vi "test_libssh2_channel_write_stderr.vi"() -> ()   [LabVIEW 2013, in "libssh2_integration_tests.lvlib"]
uses:
  libssh2_integration_tests.lvlib
  <vilib>/addons/_JKI Toolkits/Caraya/classes/Test/Test.lvclass
  libssh2/libssh2.lvlib
  <vilib>/addons/_JKI Toolkits/Caraya/classes/Assert/Assert.lvclass
panel:
  out "error out":errorcluster
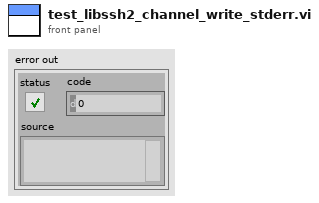
[diagram p1: front panel]
types:
  T1 = typedef "libssh2.lvlib/Session Refnum.ctl" = refnum<k1>
  T2 = typedef "libssh2.lvlib/Channel Refnum.ctl" = refnum<k1>
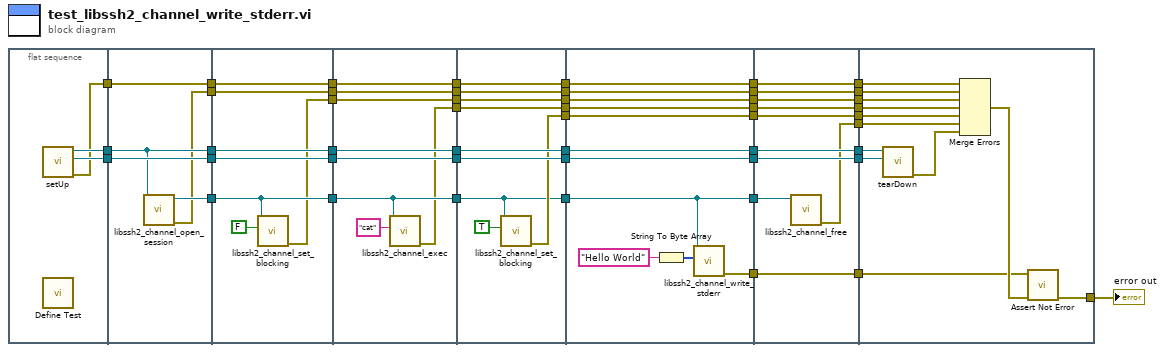
[diagram p0: block diagram]
diagram:
  n1 = flat-sequence {
    tunnel: [w51] -> w48
    tunnel: [w50] -> w47
    tunnel: [w49] -> w46
    tunnel: w48 -> [w55]
    tunnel: w47 -> [w56]
    tunnel: [w55] -> w38
    tunnel: [w56] -> w36
    tunnel: [w54] -> w30
    tunnel: w46 -> [w53]
    tunnel: [w53] -> w34
    tunnel: [w52] -> w32
    tunnel: w38 -> [w63]
    tunnel: [w63] -> w37
    tunnel: w36 -> [w62]
    tunnel: [w62] -> w35
    tunnel: w34 -> [w61]
    tunnel: [w61] -> w33
    tunnel: w32 -> [w60]
    tunnel: [w60] -> w31
    tunnel: w30 -> [w59]
    tunnel: [w59] -> w29
    tunnel: [w57] -> w28
    tunnel: w37 -> [w71]
    tunnel: [w71] -> w26
    tunnel: w35 -> [w70]
    tunnel: [w70] -> w24
    tunnel: w33 -> [w69]
    tunnel: [w69] -> w22
    tunnel: w31 -> [w68]
    tunnel: [w68] -> w20
    tunnel: w29 -> [w67]
    tunnel: [w67] -> w18
    tunnel: [w65] -> w16
    tunnel: w28 -> [w64]
    tunnel: [w64] -> w14
    tunnel: w26 -> [w80]
    tunnel: [w80] -> w25
    tunnel: w24 -> [w79]
    tunnel: [w79] -> w23
    tunnel: w22 -> [w78]
    tunnel: [w78] -> w21
    tunnel: w20 -> [w77]
    tunnel: [w77] -> w19
    tunnel: w18 -> [w72]
    tunnel: [w72] -> w17
    tunnel: w16 -> [w76]
    tunnel: [w76] -> w15
    tunnel: w14 -> [w75]
    tunnel: [w75] -> w13
    tunnel: [w73] -> w12
    tunnel: w25 -> [w91]
    tunnel: [w91] -> w9
    tunnel: w23 -> [w90]
    tunnel: [w90] -> w8
    tunnel: w21 -> [w89]
    tunnel: [w89] -> w7
    tunnel: w19 -> [w88]
    tunnel: [w88] -> w6
    tunnel: w17 -> [w87]
    tunnel: [w87] -> w5
    tunnel: w15 -> [w86]
    tunnel: [w86] -> w4
    tunnel: w13 -> [w85]
    tunnel: [w85] -> w3
    tunnel: w12 -> [w84]
    tunnel: [w84] -> w2
    tunnel: [w83] -> w1
    tunnel: w9 -> [w101]
    tunnel: w8 -> [w100]
    tunnel: [w101] -> w45
    tunnel: [w100] -> w44
    tunnel: [w99] -> w43
    tunnel: w7 -> [w98]
    tunnel: [w98] -> w42
    tunnel: w6 -> [w97]
    tunnel: [w97] -> w41
    tunnel: w5 -> [w96]
    tunnel: w4 -> [w95]
    tunnel: [w95] -> w39
    tunnel: w3 -> [w94]
    tunnel: [w94] -> w27
    tunnel: w2 -> [w93]
    tunnel: [w93] -> w11
    tunnel: [w92] -> w10
    tunnel: w1 -> [w92]
    tunnel: w45 -> [w113]
    tunnel: w44 -> [w112]
    tunnel: [w111] -> w40
    tunnel: w43 -> [w109]
    tunnel: w42 -> [w108]
    tunnel: w41 -> [w106]
    tunnel: w39 -> [w105]
    tunnel: w27 -> [w104]
    tunnel: w11 -> [w103]
    tunnel: w10 -> [w102]
    frame #0 {
      n2 = call "setUp.vi"() -> ("error out"=w49:errorcluster, "connection ID"=w50:refnum<k5>, "session"=w51:T1)  [unwired: 9 in]
      n3 = call <vilib>:"Define Test.vi"() -> ()  [unwired: 10 in, 2 out]
    }
    frame #1 {
      n4 = call "libssh2_channel_open_session.vi"("session"=w55) -> ("error out"=w52:errorcluster, "channel"=w54:T2)  [unwired: 9 in]
    }
    frame #2 {
      n5 = call "libssh2_channel_set_blocking.vi"("blocking"=FALSE, "channel"=w59) -> ("error out"=w57:errorcluster)  [unwired: 9 in]
    }
    frame #3 {
      n6 = call "libssh2_channel_exec.vi"("command"="cat", "channel"=w67) -> ("error out"=w65:errorcluster)  [unwired: 9 in]
    }
    frame #4 {
      n7 = call "libssh2_channel_set_blocking.vi"("blocking"=TRUE, "channel"=w72) -> ("error out"=w73:errorcluster)  [unwired: 9 in]
    }
    frame #5 {
      n8 = String To Byte Array(string="Hello World") -> (unsigned byte array=w82:u8[])
      n9 = call "libssh2_channel_write_stderr.vi"("buffer"=w82, "channel"=w87) -> ("error out"=w83:errorcluster)  [unwired: 8 in, 1 out]
    }
    frame #6 {
      n10 = call "libssh2_channel_free.vi"("channel"=w96) -> ("error out"=w99:errorcluster)  [unwired: 10 in]
    }
    frame #7 {
      n11 = call "tearDown.vi"("connection ID"=w112, "session"=w113) -> ("error out"=w110:errorcluster)  [unwired: 9 in]
      n12 = Merge Errors(w108, w106, w104, w105, w103, w109, w110) -> (w107:errorcluster)
      n13 = call <vilib>:"Assert Not Error.vi"("error in (no error)"=w107, "Not Error?"=w102) -> ("error out"=w111:errorcluster)  [unwired: 8 in, 1 out]
    }
  }
  "error out" <- w40
